vi "BlueTooth.Connect Test.vi"(8 "error in":errorcluster, 9 "Adapter PID":string="1015", 10 "Adapter VID":string="1366", 11 "SN":string) -> (0 "error out":errorcluster, 1 "Discovered Device":string, 2 "Result Code":i32, 3 "Success":bool, 4 "Dur(s)":dbl, 5 "STDOUT":string, 7 "Port":string)   [LabVIEW 2018]
uses:
  Utils/Errors/Error.Error Code List.ctl
panel:
  out "Cmd":string
  out "STDOUT":string
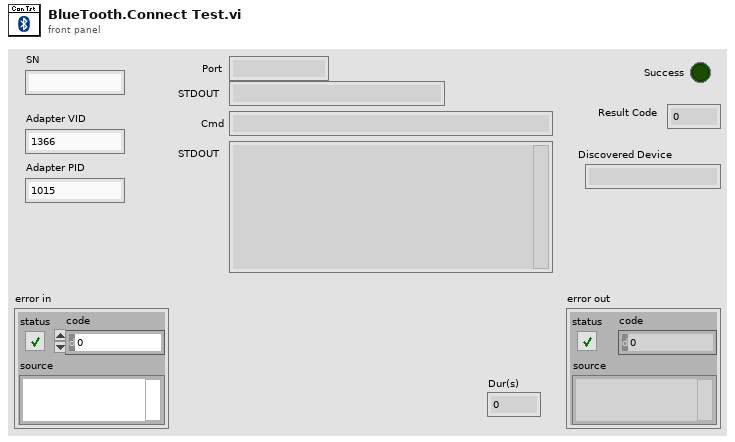
[diagram p1: front panel]
types:
  T1 = enum32{"invalid app kind", "Development System", "Run Time System", "Student Edition", "Embedded LabVIEW", "Evaluation", "Custom"}
  T2 = typedef "Error.Error Code List.ctl" = i32
  T3 = cluster{"Port":string, "Start":dbl, "Device":string, "Addr":string, "Success":bool, "Result":i32, "STDOUT":string, "Tries":i32}
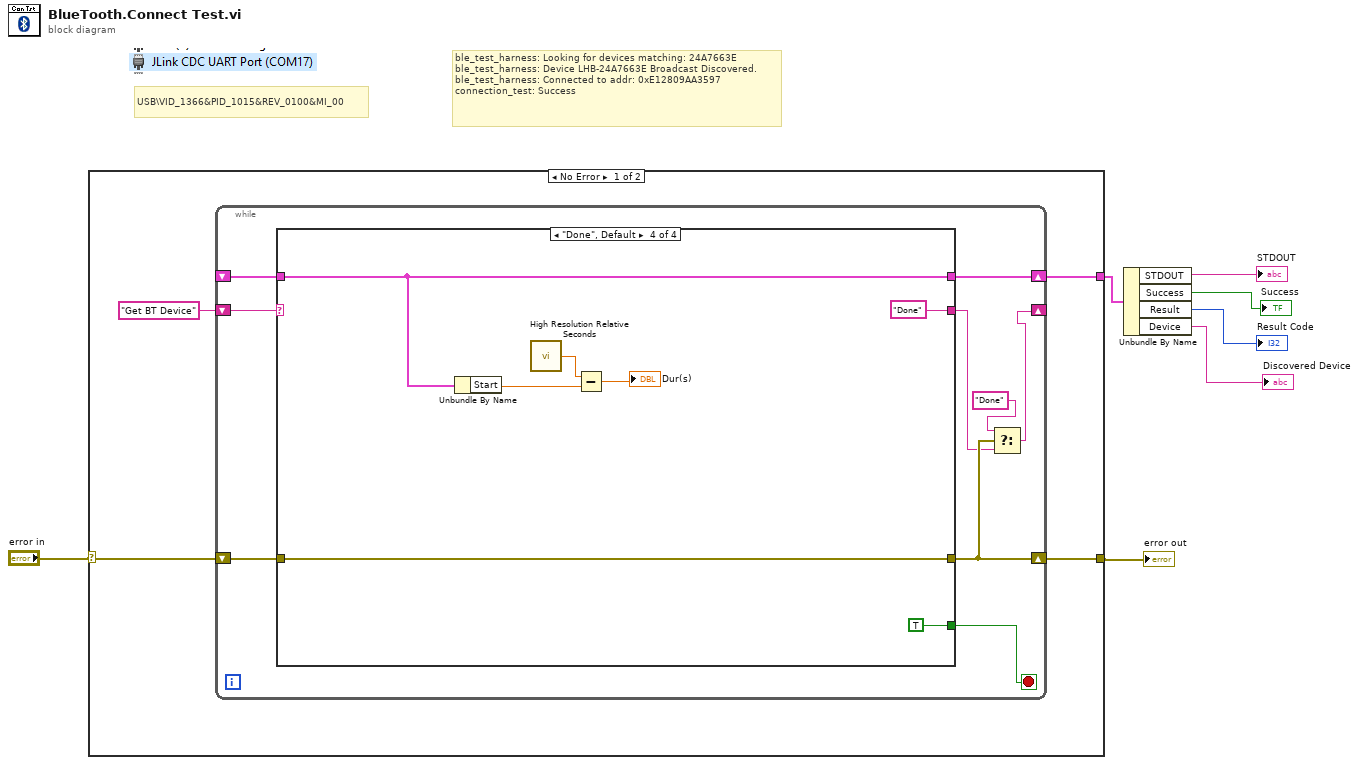
[diagram p0: block diagram]
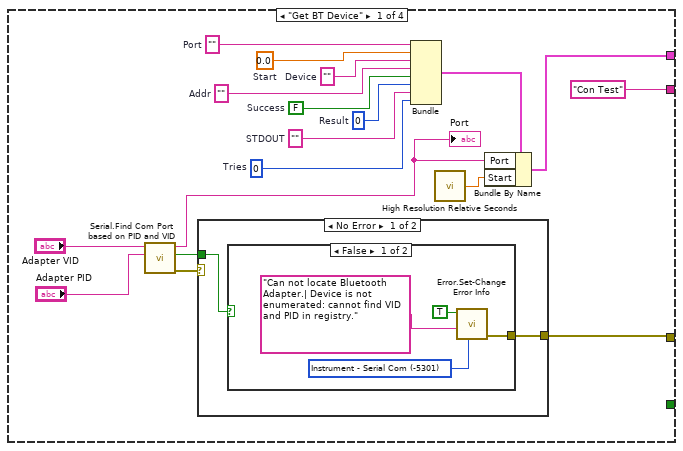
[diagram p2: hidden frame]
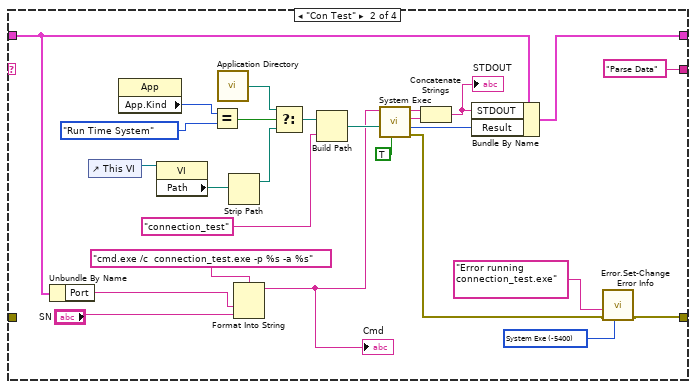
[diagram p5: hidden frame]
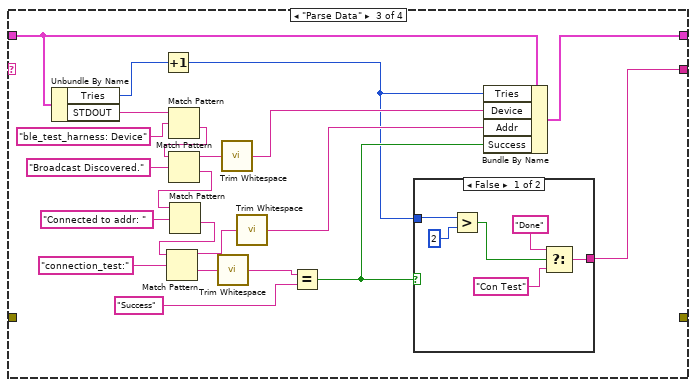
[diagram p6: hidden frame]
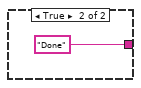
[diagram p7: hidden frame]
diagram:
  # "ble_test_harness: Looking for devices matching: 24A7663E\nble_test_harness: Device LHB-24A7663E Broadcast Discovered.\nble_test_harness: Connected to addr: 0xE12809AA3597\nconnection_test: Success"
  # "USB\\VID_1366&PID_1015&REV_0100&MI_00"
  n1 = case shown="No Error" "error in" {
    selector: "error in" -> [w10 w107]
    tunnel: [w9 w107] -> w6
    tunnel: [w8 _] -> w5
    frame No Error {
      n2 = while {
        shift-right: [w19] -> w8
        shift-left: _ -> [w18]
        shift-right: [w15] -> _
        shift-left: "Get BT Device" -> [w20]
        shift-right: [w13] -> w9
        shift-left: w10 -> [w17]
        stop <- w16 stop-if-true
        n3 = case shown="\"Done\", Default" w20 {
          tunnel: ["Con Test" "Parse Data" w72 "Done"] -> w12
          tunnel: [w25 w59 w91 w102] -> w19
          tunnel: w18 -> [_ w60 w92 w102]
          tunnel: [_ _ _ TRUE] -> w16
          tunnel: w17 -> [_ _ _ w105]
          tunnel: [w24 w49 _ w105] -> w13
          frame "Get BT Device" {
            w21 = 0  # Tries
            w23 = ""  # STDOUT
            w27 = 0  # Result
            w28 = FALSE  # Success
            w29 = ""  # Addr
            w30 = ""  # Device
            w33 = 0.0  # Start
            w34 = ""  # Port
            n4 = call "Serial.Find Com Port based on PID and VID.vi"("PID"="Adapter PID", "VID"="Adapter VID") -> ("error out"=w36:errorcluster, "Found"=w35:bool, "COM Port"=w22:string)  [unwired: 7 in]
            "Port" <- w22
            n5 = case shown="No Error" w36 {
              selector: w36 -> [_ w45]
              tunnel: w35 -> [w40 _]
              tunnel: [w39 w45] -> w24
              frame No Error {
                n6 = case shown="False" w40 {
                  tunnel: [w44 _] -> w39
                  frame False {
                    w41 = T2 -5301 items=["No Error"=0, "Abort"=-2, "Misc"=-5000, "Fixture Error"=-5100, "File IO - General"=-5200, "FIle IO - Config Error"=-5201, "Instrument - General"=-5300, "Instrument - Serial Com"=-5301, "Instrument - Camera"=-5302, "Instrument - PS"=-5303, "Instrument - Oscilloscope"=-5304, "Instrument - Function Gen"=-5305, "Instrument - Load"=-5306, "Instrument - Meter"=-5307, "Instrument - Power Control"=-5308, "Instrument - Motion"=-5309, "Instrument - RF"=-5310, "System Exe"=-5400, "Image Processing"=-5500, "Communication"=-5600, "Script - Syntax Error"=-6000, "Script - Invalid Name or Param"=-6100, "Script - Timeout"=-6200, "Invalid Data"=-6300] ("Std Code")
                    n7 = call "Error.Set-Change Error Info.vi"("Std Code"=w41, "Description"="Can not locate Bluetooth Adapter.| Device is not enumerated: cannot find VID and PID in registry.", "Set Error"=TRUE) -> ("error out"=w44:errorcluster)  [unwired: 8 in]
                  }
                  frame True {
                  }
                }
              }
              frame Error {
              }
            }
            n8 = Bundle("Port"=w34, "Start"=w33, "Device"=w30, "Addr"=w29, "Success"=w28, "Result"=w27, "STDOUT"=w23, "Tries"=w21) -> (w31:T3)  [unwired: 1 in]
            n9 = call <vilib>:"High Resolution Relative Seconds.vi"() -> ("relative seconds"=w26:dbl)
            n10 = Bundle By Name(cluster=w31, "Port"=w22, "Start"=w26) -> (w25:T3)
          }
          frame "Con Test" {
            w46 = T2 -5400 items=["No Error"=0, "Abort"=-2, "Misc"=-5000, "Fixture Error"=-5100, "File IO - General"=-5200, "FIle IO - Config Error"=-5201, "Instrument - General"=-5300, "Instrument - Serial Com"=-5301, "Instrument - Camera"=-5302, "Instrument - PS"=-5303, "Instrument - Oscilloscope"=-5304, "Instrument - Function Gen"=-5305, "Instrument - Load"=-5306, "Instrument - Meter"=-5307, "Instrument - Power Control"=-5308, "Instrument - Motion"=-5309, "Instrument - RF"=-5310, "System Exe"=-5400, "Image Processing"=-5500, "Communication"=-5600, "Script - Syntax Error"=-6000, "Script - Invalid Name or Param"=-6100, "Script - Timeout"=-6200, "Invalid Data"=-6300] ("Std Code")
            n11 = Unbundle By Name(w60) -> ("Port"=w56:string)
            n12 = control-ref of="This VI"() -> (w65:refnum<vi>)
            n13 = property class="App"() -> ("App.Kind"=w64:T1)  [unwired: 2 in, 2 out]
            n14 = property class="VI"(reference=w65) -> ("Path"=w66:path)  [unwired: 1 in, 2 out]
            n15 = Equal?(x=w64, y=T1."Run Time System" ("Application:Kind")) -> (x = y?=w67:bool)
            n16 = call <vilib>:"Application Directory.vi"() -> ("Application Directory"=w68:path)
            n17 = Strip Path(path=w66) -> (stripped path=w69:path)  [unwired: 1 out]
            n18 = Format Into String(format string="cmd.exe /c  connection_test.exe -p %s -a %s", w56, "SN") -> (resulting string=w53:string)  [unwired: 2 in, 1 out]
            "Cmd" <- w53
            n19 = Select(t=w68, s=w67, f=w69) -> (s? t:f=w70:path)
            n20 = Build Path(base path=w70, name or relative path="connection_test") -> (appended path=w71:path)
            n21 = call <vilib>:"System Exec.vi"("run minimized? (F)"=TRUE, "working directory"=w71, "command line"=w53) -> ("error out"=w48:errorcluster, "return code"=w58:i32, "standard error"=w51:string, "standard output"=w52:string)  [unwired: 5 in]
            n22 = Concatenate Strings(w52, w51) -> (w50:string)
            "STDOUT" <- w50
            n23 = Bundle By Name(cluster=w60, "STDOUT"=w50, "Result"=w58) -> (w59:T3)
            n24 = call "Error.Set-Change Error Info.vi"("Std Code"=w46, "error in"=w48, "Description"="Error running connection_test.exe") -> ("error out"=w49:errorcluster)  [unwired: 8 in]
          }
          frame "Parse Data" {
            n25 = Unbundle By Name(w92) -> ("Tries"=w75:i32, "STDOUT"=w90:string)
            n26 = Increment(x=w75) -> (x+1=w73:i32)
            n27 = Match Pattern(string=w90, regular expression="ble_test_harness: Device" ("Device")) -> (after substring=w88:string)  [unwired: 1 in, 3 out]
            n28 = Match Pattern(string=w88, regular expression="Broadcast Discovered." ("Device")) -> (before substring=w86:string, after substring=w84:string)  [unwired: 1 in, 2 out]
            n29 = Match Pattern(string=w84, regular expression="Connected to addr: " ("Device")) -> (after substring=w83:string)  [unwired: 1 in, 3 out]
            n30 = Match Pattern(string=w83, regular expression="connection_test:" ("Device")) -> (before substring=w80:string, after substring=w81:string)  [unwired: 1 in, 2 out]
            n31 = call <vilib>:"Trim Whitespace.vi"("string"=w81) -> ("trimmed string"=w77:string)  [unwired: 1 in]
            n32 = call <vilib>:"Trim Whitespace.vi"("string"=w86) -> ("trimmed string"=w79:string)  [unwired: 1 in]
            n33 = call <vilib>:"Trim Whitespace.vi"("string"=w80) -> ("trimmed string"=w78:string)  [unwired: 1 in]
            n34 = Equal?(x=w77, y="Success" ("Device")) -> (x = y?=w74:bool)
            n35 = case shown="False" w74 {
              tunnel: w73 -> [w98 _]
              tunnel: [w96 "Done"] -> w72
              frame False {
                n36 = Greater?(x=w98, y=2) -> (0:w95:bool)
                n37 = Select(t="Done", s=w95, f="Con Test") -> (s? t:f=w96:string)
              }
              frame True {
              }
            }
            n38 = Bundle By Name(cluster=w92, "Tries"=w73, "Device"=w79, "Addr"=w78, "Success"=w74) -> (w91:T3)
          }
          frame "Done", Default {
            n39 = Unbundle By Name(w102) -> ("Start"=w101:dbl)
            n40 = call <vilib>:"High Resolution Relative Seconds.vi"() -> ("relative seconds"=w104:dbl)
            n41 = Subtract(x=w104, y=w101) -> (x-y=→"Dur(s)":dbl)
          }
        }
        n42 = Select(t="Done", s=w13, f=w12) -> (s? t:f=w15:string)
      }
    }
    frame Error {
    }
  }
  "error out" <- w6
  n43 = Unbundle By Name(w5) -> ("STDOUT"=→"STDOUT":string, "Success"=→"Success":bool, "Result"=→"Result Code":i32, "Device"=→"Discovered Device":string)
